vi "rql_Create Read Worker.vi"(4 "Show in Debugger?":bool=TRUE, 6 "Message Priority":T1=enum."Normal", 8 "error in":errorcluster, 9 "Data in":T2={"Forwarding Q"=refnum, "DC_UID"="", "Worker Alias"="", "Message Priority"=enum."Normal"}, 11 "DS TCP Server in":refnum<class "DS TCP Server.lvclass">) -> (0 "error out":errorcluster, 3 "dup DS TCP Server out":refnum<class "DS TCP Server.lvclass">)   [LabVIEW 2017, in "DS TCP Server.lvlib" / "DS TCP Server.lvclass"]
doc: "This VI sends a <b>Local API Request</b> message to an MHL case of the Worker that owns this VI.\n---\nLaunch a TCP Read Worker to receive incoming data from a Debug Client"
uses:
  DS TCP Server.lvclass
  C:/Program Files (x86)/National Instruments/LabVIEW 2017/vi.lib/addons/_Workers/Library/Classes/Worker/Worker.lvclass
  rql_Create Read Worker.ctl
  <vilib>/addons/_Workers/Library/Classes/Message Queue/Message Queue.lvclass
  Common VIs/DC_UID.ctl
  <vilib>/addons/_Workers/Library/Classes/Message/Priority.ctl
  <vilib>/addons/_Workers/Library/Classes/Worker/Worker.lvclass/Worker.ctl
  <vilib>/addons/_Workers/Library/Classes/Worker/Worker.lvclass
  <vilib>/addons/_Workers/Library/Classes/Message/Message.lvclass
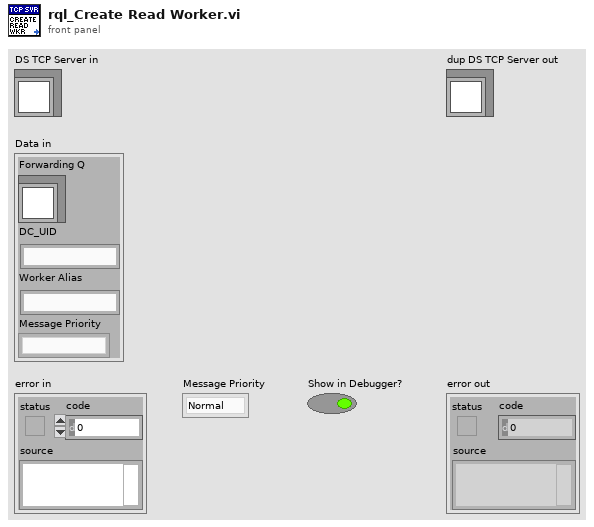
[diagram p1: front panel]
types:
  T1 = typedef "Workers.lvlib/Message.lvclass/Priority.ctl" = enum16{"Low", "Normal", "High"}
  T2 = typedef "DS TCP Server.lvlib/DS TCP Server.lvclass/rql_Create Read Worker.ctl" = cluster{"Forwarding Q":refnum<class "Message Queue.lvclass">, "DC_UID":T3, "Worker Alias":string, "Message Priority":T1}
  T3 = typedef "DC_UID.ctl" = string
  T4 = typedef "Workers.lvlib/Case Label.ctl" = string
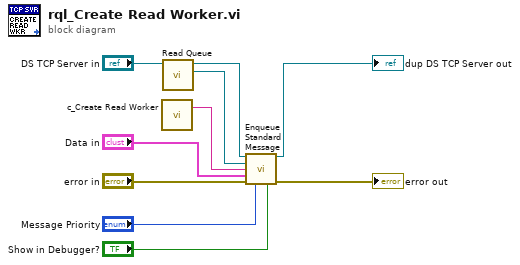
[diagram p0: block diagram]
diagram:
  n1 = call "c_Create Read Worker.vi"() -> ("Case Label"=w4:T4)  [unwired: 1 in]
  n2 = call <vilib>:"Read Queue.vi"("Worker_"="DS TCP Server in") -> ("Message Queue out"=w5:refnum<class "Message Queue.lvclass">, "dup Worker_out"=w6:refnum<class "DS TCP Server.lvclass">)  [unwired: 9 in]
  n3 = call-dynamic "Enqueue Standard Message.vi"("Worker"=w6, "Message Queue"=w5, "Case Label"=w4, "Data"="Data in", "error in (no error)"="error in", "Priority (Normal)"="Message Priority", "Send Message to Debugger? (T)"="Show in Debugger?") -> ("dup Worker out"=→"dup DS TCP Server out":refnum<class "DS TCP Server.lvclass">, "error out"=→"error out":errorcluster)  [unwired: 7 in]
